vi "SubVI_IntakeWheels_teleop.vi"(6 "teleop/auto":bool, 9 "auto speed":dbl=0.9 format="%#_13g", 10 "SpitCube":bool, 11 "TakeInCube":bool) -> ()   [LabVIEW 2017]
panel:
  in  "intake out":dbl=0.9 format="%#_13g"
  in  "intake in":dbl=-0.6 format="%#_13g"
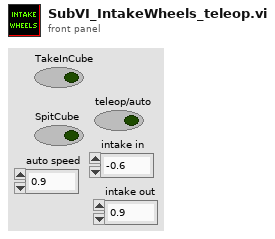
[diagram p1: front panel]
types:
  T1 = typedef "WPI_MotorControlDeviceRef.ctl" = cluster{"DeviceStatus":errorcluster, "Type":T2, "PWM":cluster{"PWM Channel":T3, "DeadBand":T4}, "CAN":cluster{"Device Number":u8, "SetOutput VI Ref":variant, "GetOutput VI Ref":variant, "Enable VI Ref":variant, "Disable VI Ref":variant, "Data":variant}, "Invert":bool, "DIO PWM":cluster{"PWM \"Enable\" Channel":T3, "DIOChannel":T5, "PWM Rate":dbl}}
  T2 = typedef "WPI_MotorControlType.ctl" = enum16{"PWM", "CAN", "DIO PWM"}
  T3 = typedef "FPGA_DIOPWMChannel.ctl" = enum8{"PWM 0", "PWM 1", "PWM 2", "PWM 3", "PWM 4", "PWM 5", "PWM 6", "PWM 7", "PWM 8", "PWM 9", "PWM MXP 0", "PWM MXP 1", "PWM MXP 2", "PWM MXP 3", "PWM MXP 4", "PWM MXP 5", "PWM MXP 6", "PWM MXP 7", "PWM MXP 8", "PWM MXP 9", "Invalid"}
  T4 = typedef "WPI_PWMDeadband.ctl" = cluster{"Name":string, "maxPositivePwm":i32, "minPositivePwm":i32, "centerPwm":i32, "maxNegativePwm":i32, "minNegativePwm":i32, "angularRange":u16}
  T5 = typedef "FPGA_DIOChannel.ctl" = enum8{"DIO 0", "DIO 1", "DIO 2", "DIO 3", "DIO 4", "DIO 5", "DIO 6", "DIO 7", "DIO 8", "DIO 9", "DIO MXP 0", "DIO MXP 1", "DIO MXP 2", "DIO MXP 3", "DIO MXP 4", "DIO MXP 5", "DIO MXP 6", "DIO MXP 7", "DIO MXP 8", "DIO MXP 9", "DIO MXP 10", "DIO MXP 11", "DIO MXP 12", "DIO MXP 13", "DIO MXP 14", "DIO MXP 15", "SPI Port CS1", "SPI Port CS2", "SPI Port CS3", "SPI Port MISO", "SPI Port MOSI", "Invalid"}
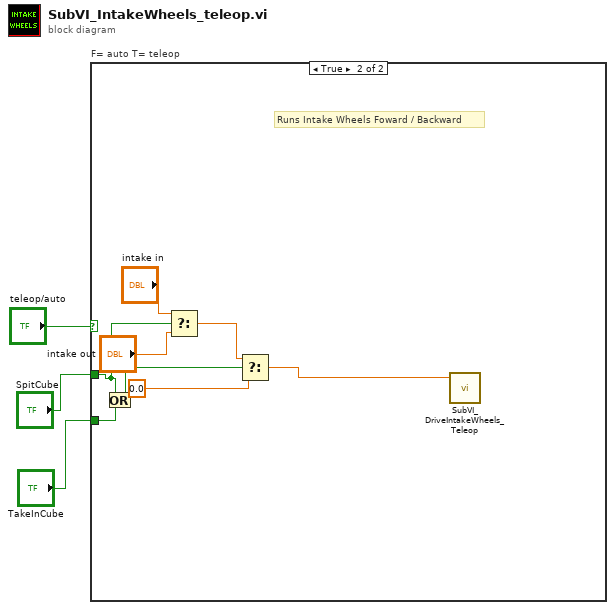
[diagram p0: block diagram]
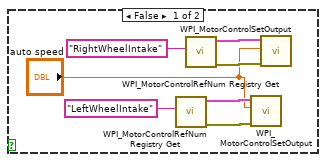
[diagram p2: hidden frame]
diagram:
  n1 = case "F= auto T= teleop" shown="True" "teleop/auto" {
    tunnel: "SpitCube" -> [_ w13]
    tunnel: "TakeInCube" -> [_ w15]
    frame False {
      n2 = call <vilib>:"WPI_MotorControlRefNum Registry Get.vi"("refnum name"="LeftWheelIntake") -> ("error out"=w7:errorcluster, "MotorControlDevRef"=w9:T1)  [unwired: 9 in]
      n3 = call <vilib>:"WPI_MotorControlRefNum Registry Get.vi"("refnum name"="RightWheelIntake") -> ("error out"=w8:errorcluster, "MotorControlDevRef"=w10:T1)  [unwired: 9 in]
      n4 = call <vilib>:"WPI_MotorControlSetOutput.vi"("error in (no error)"=w7, "Output"="auto speed", "MotorControlDevRef"=w9) -> ()  [unwired: 6 in, 3 out]
      n5 = call <vilib>:"WPI_MotorControlSetOutput.vi"("error in (no error)"=w8, "Output"="auto speed", "MotorControlDevRef"=w10) -> ()  [unwired: 6 in, 3 out]
    }
    frame True {
      # "Runs Intake Wheels Foward / Backward"
      n6 = Or(x=w13, y=w15) -> (x .or. y?=w17:bool)
      n7 = Select(t="intake in", s=w13, f="intake out") -> (s? t:f=w14:dbl)
      n8 = Select(t=w14, s=w17, f=0.0) -> (s? t:f=w18:dbl)
      n9 = call "SubVI_DriveIntakeWheels_Teleop.vi"("speed"=w18) -> ()  [unwired: 11 in]
    }
  }
